vi "SIStapelFFT.vi"() -> ()   [LabVIEW 2011]
uses:
  <vilib>/Analysis/2dsp.llb/2D Cross Correlation (DBL).vi
  <vilib>/Analysis/2dsp.llb/2D Complex FFT.vi
  <vilib>/Analysis/NI_AALPro.lvlib
  <vilib>/Analysis/NI_AALBase.lvlib
panel:
  out "Numeric":i32
  in  "~Peek":i32[](array[numeric])=[82, 234]
  out "Intensity Graph 3":dbl[][](graph)
  in  "index (pageN)":i32=1
  out "cross corr":dbl[][](graph)
  out "x*y":dbl
  out "slope":dbl
  out "Grid-Angle-To ImageAxis (~19°)":dbl format="%0.2f"
  out "Pitch":dbl
  out "Intensity Graph 2":dbl[][](graph)
  out "max index(es)":i32[](array[numeric])
  out "Amplitude":dbl[](graph)
  out "Phaseshift":dbl[](graph)
  out "pageN-0":i16[][](graph)
  out "Intensity Graph":dbl[][](graph)
  out "crop size(s)":i32[](array[numeric])
  out "size(s)":i32[](array[numeric])
  in  "file path":path
  # "sipcharts-raw"
  # "muss +-15 passen!"
  # "29gitter 72/205\n25gitter 82/233"
  # "flumias 65/74"
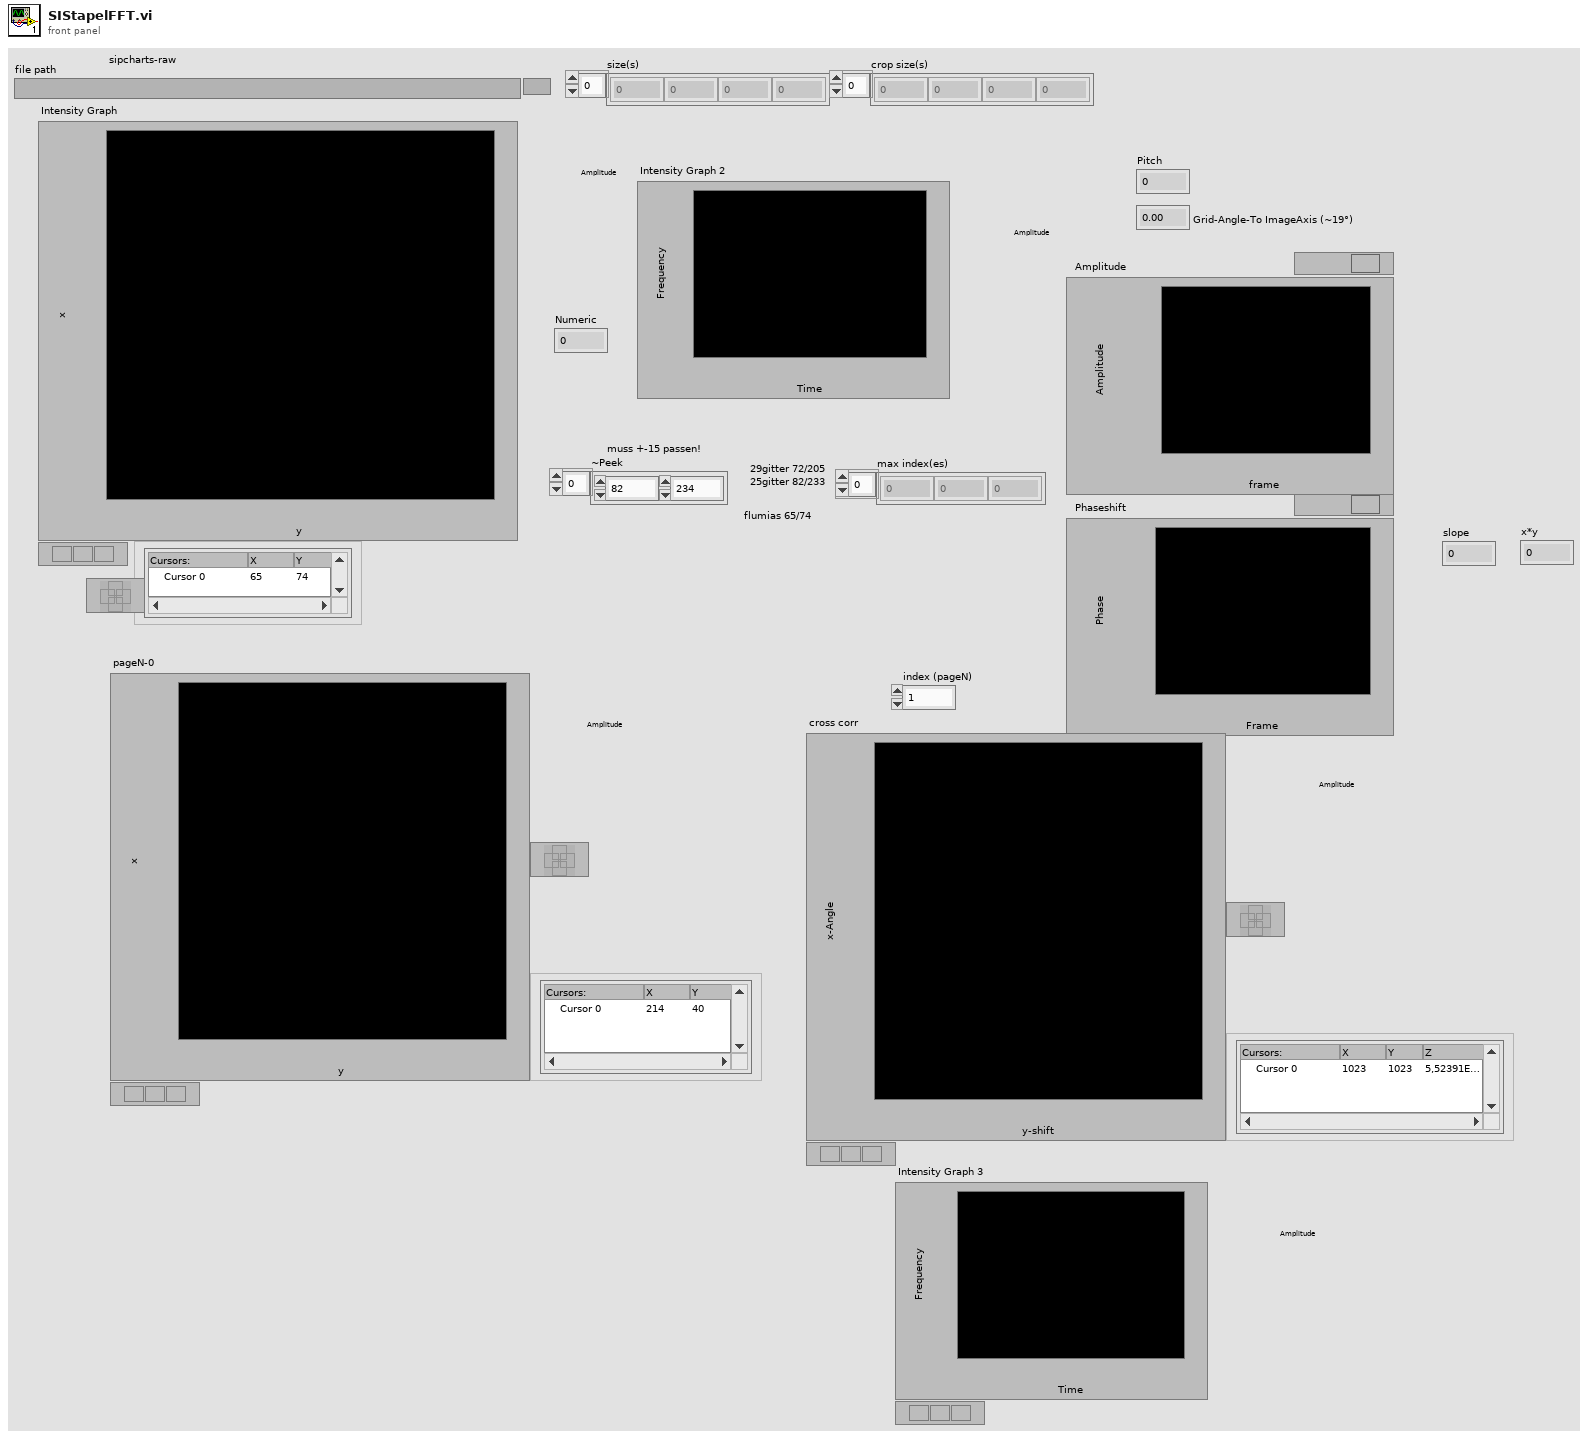
[diagram p1: front panel]
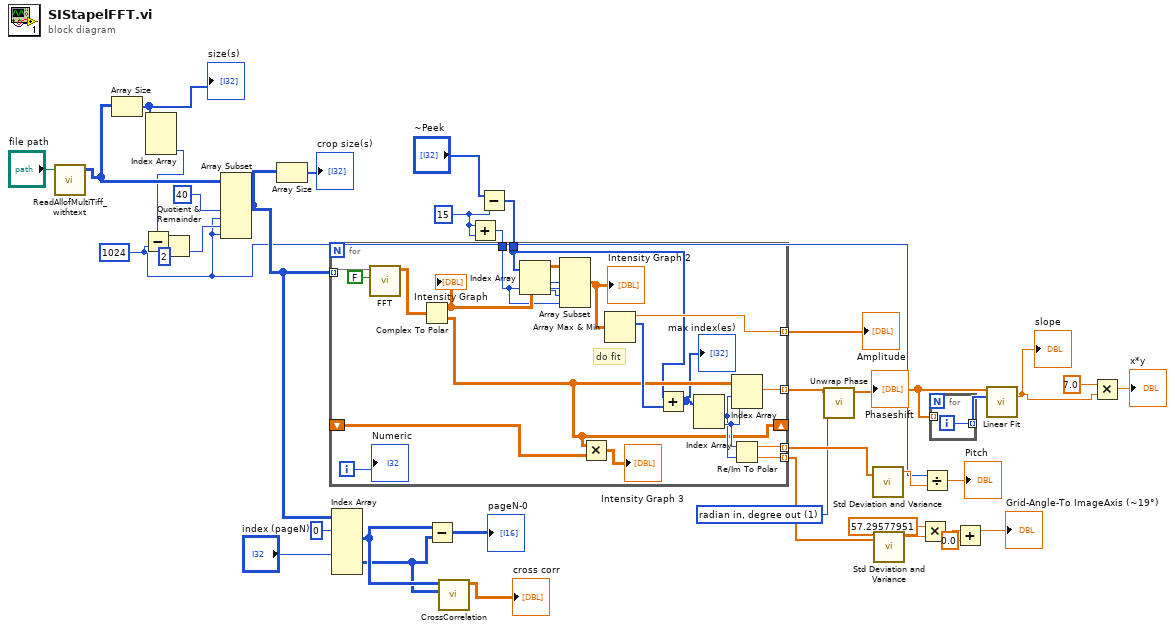
[diagram p0: block diagram]
diagram:
  w2 = 1 items=["radian in, radian out", "radian in, degree out", "degree in, degree out", "degree in, radian out"] ("phase unit")
  w22 = 15 ("length")
  w17 = 1024 ("m")
  n1 = call "ReadAllofMultiTiff_withtext.vi"("file path"="file path") -> ("16-bit pixmaps"=w37:i16[][][])  [unwired: 2 in, 2 out]
  n2 = Array Size(array=w37) -> (size(s)=w34:i32[])
  "size(s)" <- w34
  n3 = Index Array(array=w34) -> (element #3=w33:i32)  [unwired: 3 in, 2 out]
  n4 = Subtract(x=w33, y=w17) -> (x-y=w32:i32)
  n5 = Quotient & Remainder(x=w32, y=2) -> (floor(x/y)=w30:i32)  [unwired: 1 out]
  n6 = Array Subset(array=w37, index (dim 1)=40 ("index"), length (dim 1)=w17, index (dim 2)=w30, length (dim 2)=w17) -> (w29:i16[][][])  [unwired: 2 in]
  n7 = Array Size(array=w29) -> (size(s)=→"crop size(s)":i32[])
  n8 = Index Array(array=w29, index (dim 0) #1=0 ("index (page)"), index (dim 0) #2="index (pageN)") -> (element #1=w25:i16[][], element #2=w24:i16[][])  [unwired: 4 in]
  n9 = Subtract(x=w25, y=w24) -> (x-y=→"pageN-0":i16[][])
  n10 = call-poly <vilib>:"CrossCorrelation.vi"("Y"=w24, "X"=w25) -> ("Rxy"=→"cross corr":dbl[][])  [unwired: 8 in, 1 out]
  n11 = Add(x=w22, y=w22) -> (x+y=w21:i32)
  n12 = Subtract(x="~Peek", y=w22) -> (x-y=w23:i32[])
  n13 = for {
    tunnel: w29 -> [w59] mode=indexing
    tunnel: [w56] -> w9 mode=indexing
    tunnel: w23 -> [w41]
    tunnel: w21 -> [w54]
    tunnel: [w53] -> w20 mode=indexing
    tunnel: [w48] -> w15 mode=indexing
    tunnel: [w47] -> w10 mode=indexing
    shift-right: [w44] -> _
    shift-left: _ -> [w43]
    i -> [w39]
    # "do fit"
    n14 = call-poly <vilib>:"FFT.vi"("shift?"=FALSE, "X"=w59) -> ("FFT {X}"=w57:cdb[][])  [unwired: 8 in, 1 out]
    n15 = Complex To Polar(r * e^(i*theta)=w57) -> (r=w55:dbl[][], theta=w44:dbl[][])
    "Intensity Graph" <- w55
    n16 = Index Array(array=w41) -> (element #1=w52:i32, element #2=w51:i32)  [unwired: 2 in]
    n17 = Array Subset(array=w55, index (row)=w52, length (row)=w54, index (col)=w51, length (col)=w54) -> (w49:dbl[][])
    "Intensity Graph 2" <- w49
    n18 = Multiply(x=w44, y=w43) -> (x*y=→"Intensity Graph 3":dbl[][])
    n19 = Array Max & Min(array=w49) -> (max value=w53:dbl, max index (indices)=w50:i32[])  [unwired: 2 out]
    n20 = Add(x=w41, y=w50) -> (x+y=w40:i32[])
    "max index(es)" <- w40
    n21 = Index Array(array=w40) -> (element #1=w45:i32, element #2=w46:i32)  [unwired: 2 in]
    n22 = Index Array(array=w44, index (row)=w45, index (col)=w46) -> (element=w56:dbl)
    n23 = Re/Im To Polar(2:w45, 3:w46) -> (0:w48:dbl, 1:w47:dbl)
    "Numeric" <- w39
  }
  "Amplitude" <- w20
  n24 = call <vilib>:"Unwrap Phase.vi"("phase unit"=w2, "Phase"=w9) -> ("Unwrapped Phase"=w6:dbl[])  [unwired: 8 in, 1 out]
  "Phaseshift" <- w6
  n25 = call <vilib>:"Std Deviation and Variance.vi"("X"=w10) -> ("mean"=w18:dbl)  [unwired: 1 in, 2 out]
  n26 = call <vilib>:"Std Deviation and Variance.vi"("X"=w15) -> ("mean"=w14:dbl)  [unwired: 1 in, 2 out]
  n27 = Multiply(x=57.29577951, y=w14) -> (x*y=w12:dbl)
  n28 = Divide(x=w17, y=w18) -> (x/y=→"Pitch":dbl)
  n29 = for {
    tunnel: [w60] -> w7 mode=indexing
    tunnel: w6 -> [_] mode=indexing
    i -> [w60]
  }
  n30 = Add(x=w12, y=0.0) -> (x+y=→"Grid-Angle-To ImageAxis (~19°)":dbl)
  n31 = call <vilib>:"Linear Fit.vi"("Y"=w6, "X"=w7) -> ("slope"=w1:dbl)  [unwired: 9 in, 4 out]
  "slope" <- w1
  n32 = Multiply(x=7.0, y=w1) -> (x*y=→"x*y":dbl)
